vi "Voltage and Current Ring Chooser.vi"(8 "error in (no error)":errorcluster, 11 "Yokogawa WT500 in":refnum<class "Yokogawa WT500.lvclass">) -> (0 "error out":errorcluster, 3 "Yokogawa WT500 out":refnum<class "Yokogawa WT500.lvclass">)   [LabVIEW 2016, in "Generic Power Analyzer.lvlib" / "Yokogawa WT500.lvlib" / "Yokogawa WT500.lvclass"]
uses:
  Yokogawa WT500.lvclass
panel:
  in  "Voltage Range (8: 1000V)":u16(ring)=8 items=["AUTO", "15", "30", "60", "100", "150", "300", "600", "1000", "7.5", "15", "30", "50", "75", "150", "300", "500"]
  in  "Current Range (7: 40A)":u16(ring)=7 items=["AUTO", "500 mA", "1 A", "2 A", "5 A", "10 A", "20 A", "40 A", "S-AUTO", "50 mV", "100 mV", "200 mV", "500 mV", "1 V", "2 V", "5 V", "10 V", "250 mA", "500 mA", "1 A", "2.5 A", "5 A", "10 A", "20 A", "25 mV", "50 mV", "100 mV", "250 mV", "500 mV", "1 V", "2.5 V", "5 V"]
  in  "Wiring (0: 1P2W, 1P2W, 1P2W)":u16(ring) items=["1P2W, 1P2W, 1P2W", "1P3W, 1P2W", "3P3W, 1P2W", "1P2W, 1P3W", "1P2W, 3P3W", "3P4W", "3V3A"]
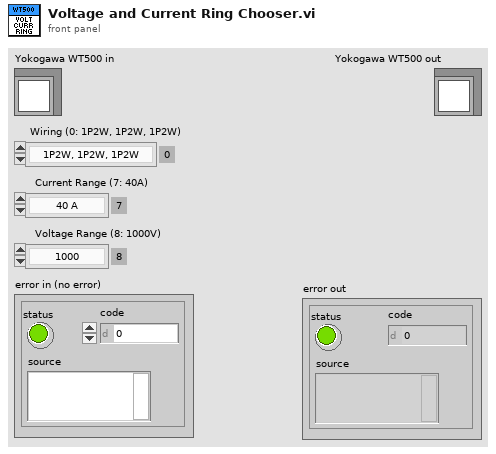
[diagram p1: front panel]
types:
  T1 = typedef "LVStringsAndValuesArrayTypeDef_U16.ctl" = cluster{"String":string, "Value":u16}[]
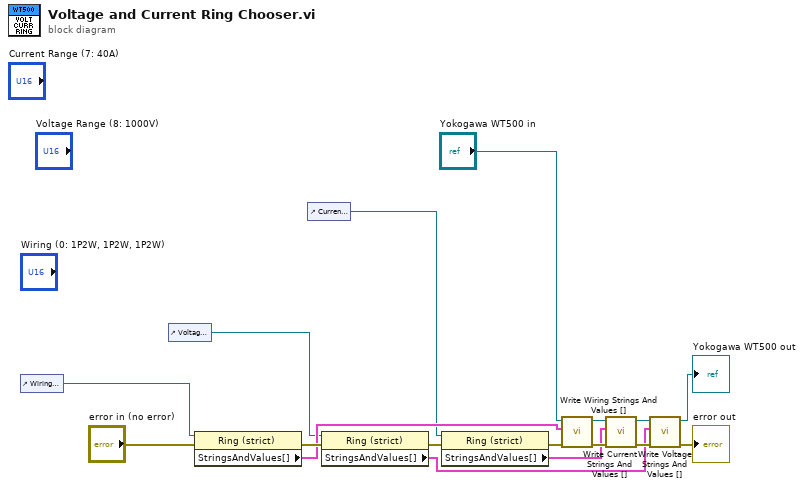
[diagram p0: block diagram]
diagram:
  n1 = control-ref of="Wiring (0: 1P2W, 1P2W, 1P2W)"() -> (w3:refnum<vi>)
  n2 = control-ref of="Voltage Range (8: 1000V)"() -> (w2:refnum<vi>)
  n3 = property class="Ring (strict)"(reference=w3, error in="error in (no error)") -> (error out=w13:errorcluster, "StringsAndValues[]"=w10:T1)  [unwired: 1 out]
  n4 = control-ref of="Current Range (7: 40A)"() -> (w1:refnum<vi>)
  n5 = property class="Ring (strict)"(reference=w2, error in=w13) -> (error out=w12:errorcluster, "StringsAndValues[]"=w9:T1)  [unwired: 1 out]
  n6 = property class="Ring (strict)"(reference=w1, error in=w12) -> (error out=w11:errorcluster, "StringsAndValues[]"=w8:T1)  [unwired: 1 out]
  n7 = call-dynamic "Write Wiring Strings And Values [].vi"("error in (no error)"=w11, "Strings And Values []"=w10, "Generic Power Analyzer in"="Yokogawa WT500 in") -> ("error out"=w15:errorcluster, "Generic Power Analyzer out"=w17:refnum<class "Yokogawa WT500.lvclass">)  [unwired: 7 in]
  n8 = call-dynamic "Write Current Strings And Values [].vi"("error in (no error)"=w15, "Strings And Values []"=w8, "Generic Power Analyzer in"=w17) -> ("error out"=w14:errorcluster, "Generic Power Analyzer out"=w16:refnum<class "Yokogawa WT500.lvclass">)  [unwired: 7 in]
  n9 = call-dynamic "Write Voltage Strings And Values [].vi"("error in (no error)"=w14, "Strings And Values []"=w9, "Generic Power Analyzer in"=w16) -> ("error out"=→"error out":errorcluster, "Generic Power Analyzer out"=→"Yokogawa WT500 out":refnum<class "Yokogawa WT500.lvclass">)  [unwired: 7 in]
